vi "Read Toggle Key Binding.vi"(8 "error in (no error)":errorcluster, 11 "MixedCheckbox.lvclass in":refnum<class "MixedCheckbox.lvclass">) -> (0 "error out":errorcluster, 2 "ToggleKeyBind":T1, 3 "MixedCheckbox.lvclass out":refnum<class "MixedCheckbox.lvclass">)   [LabVIEW 2015, in "MixedCheckbox.lvclass"]
uses:
  MixedCheckbox.lvclass
  <vilib>/Utility/miscctls.llb/LVKeyTypeDef.ctl
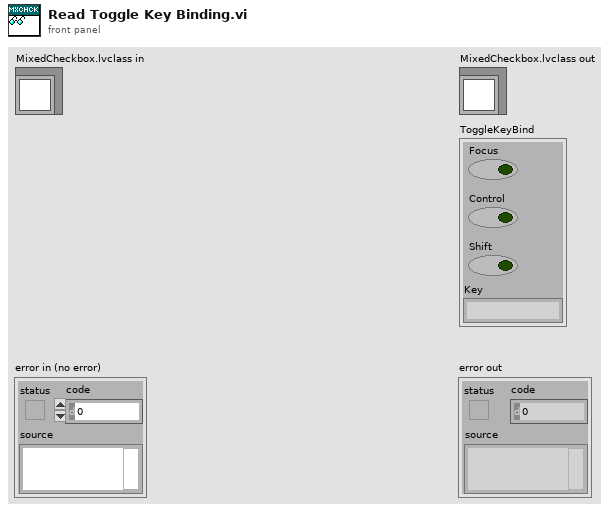
[diagram p1: front panel]
types:
  T1 = typedef "LVKeyTypeDef.ctl" = cluster{"Focus":bool, "Control":bool, "Shift":bool, "Key":string}
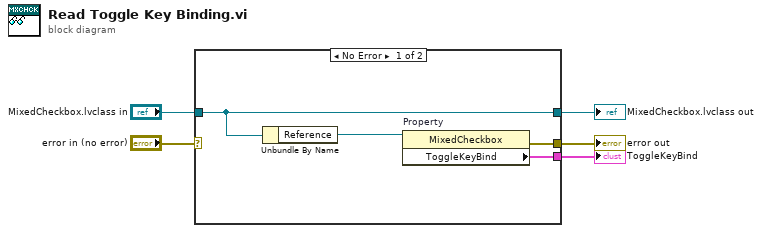
[diagram p0: block diagram]
diagram:
  n1 = case shown="No Error" "error in (no error)" {
    selector: "error in (no error)" -> [_ w11]
    tunnel: [w8 w11] -> w4
    tunnel: [w7 w10] -> w2
    tunnel: "MixedCheckbox.lvclass in" -> [w7 w10]
    tunnel: [w9 _] -> w1
    frame No Error {
      n2 = Unbundle By Name(w7) -> ("Reference"=w6:refnum<vi>)
      n3 = property on="Property" class="MixedCheckbox"(reference=w6) -> (error out=w8:errorcluster, "ToggleKeyBind"=w9:T1)  [unwired: 1 in, 1 out]
    }
    frame Error {
    }
  }
  "error out" <- w4
  "MixedCheckbox.lvclass out" <- w2
  "ToggleKeyBind" <- w1
